vi "range.vi"(3 "every":i32=1, 4 "to":i32, 5 "from":i32) -> (1 "Range":i64[](array[numeric]))   [LabVIEW 2009]
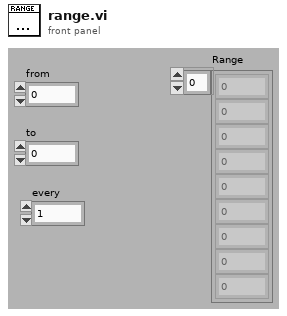
[diagram p1: front panel]
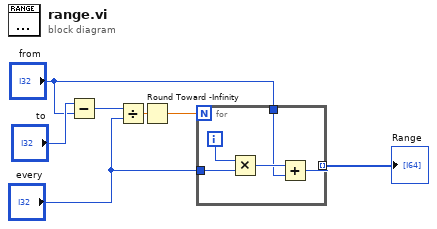
[diagram p0: block diagram]
diagram:
  n1 = Subtract(x="to", y="from") -> (x-y=w6:i32)
  n2 = Divide(x=w6, y="every") -> (x/y=w5:dbl)
  n3 = Round Toward -Infinity(1:w5) -> (0:w4:dbl)
  n4 = for {
    N: w4 -> [_]
    tunnel: "every" -> [w11]
    tunnel: [w9] -> w2 mode=indexing
    tunnel: "from" -> [w8]
    i -> [w12]
    n5 = Multiply(x=w12, y=w11) -> (x*y=w10:i32)
    n6 = Add(x=w10, y=w8) -> (x+y=w9:i32)
  }
  "Range" <- w2
